vi "WinBOOL.vi"() -> ()   [LabVIEW 2023]
doc: "This function inverts the value of input and returns it in output.\n\nFor information on the data types used for the DLL function, right-click on the Call Library Function node and choose Configure."
uses:
  CLF_Example.dll
panel:
  out "output":bool
  in  "input":bool
  # "See the block diagram for more information."
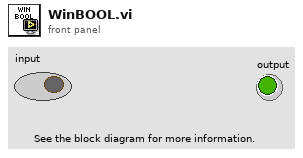
[diagram p1: front panel]
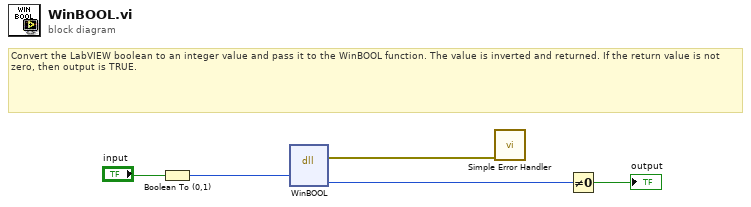
[diagram p0: block diagram]
diagram:
  # "Convert the LabVIEW boolean to an integer value and pass it to the WinBOOL function. The value is inverted and returned. If the return value is not zero, then output is TRUE."
  n1 = Boolean To (0,1)(Boolean="input") -> (0, 1=w5:i16)
  n2 = dll-call lib="c:/dev/_r/4/eng/lv-core/lvpostprocessingd/lv_mc_x86_64/dist_i386/examples/Connectivity/Libraries and Executables/DLL Calling VIs/CLF_Example**.*" fn="WinBOOL"("input"=w5) -> (error out=w1:errorcluster, "output"=w2:i32)  [unwired: 3 in, 4 out]
  n3 = call <vilib>:"Simple Error Handler.vi"("error in (no error)"=w1) -> ()  [unwired: 4 in, 5 out]
  n4 = Not Equal To 0?(x=w2) -> (x != 0?=→"output":bool)
